vi "子VI-查看某框-不显示界面-只读穿透图模式.vi"(0 "框号":dbl format="%#_13g", 1 "框组":T3(array[cluster]), 2 "临界Z值":i32, 4 "临界面积百分比值":dbl, 5 "预先配置的灰度阈值":dbl, 6 "穿透图原始路径":path, 7 "部位信息":string[](array[string])=["", "34.500000", "32.500000", "1121", "34", "54.955926", "分层类", "不合格", ""], 12 "产品规格":cluster{"产品长度（周长）（mm）":dbl, "产品宽度（母线长）（mm）":dbl}) -> (17 "全部检测结果":string[][](table))   [LabVIEW 2018]
uses:
  <vilib>/vision/NI_Vision_Development_Module.lvlib
panel:
  out "?":string[][](table)
  out "弥散类检测结果":string[][](table)
  in  "格式字符串 4":string="%f"
  in  "分隔符（'\\'代码显示） 3":string="\t"
  in  "Tab Control":T1
  out "?":T2(plugin-control)
  out "Threshold Image":T2(plugin-control)
  out "Threshold Image":T2(plugin-control)
  in  "格式字符串 3":string="%f"
  in  "分隔符（'\\'代码显示） 2":string="\t"
  out "弥散和分层临界灰度值":i64
  out "弥散缺陷个数":i32
  out "分层缺陷个数":i32
  out "合格？ 弥散类":string="fencengThreshold"
  out "合格？分层类":string="fencengThreshold"
  out "弥散测量结果":i16[][](array[numeric])
  out "面积 (pixels)":i32
  in  "格式字符串 2":string="%f"
  in  "分隔符（'\\'代码显示）":string="\t"
  out "分层测量结果":i16[][](array[numeric])
  out "缺陷初步分类的临界值":sgl format="%#.3f"
  # "所选区域信息"
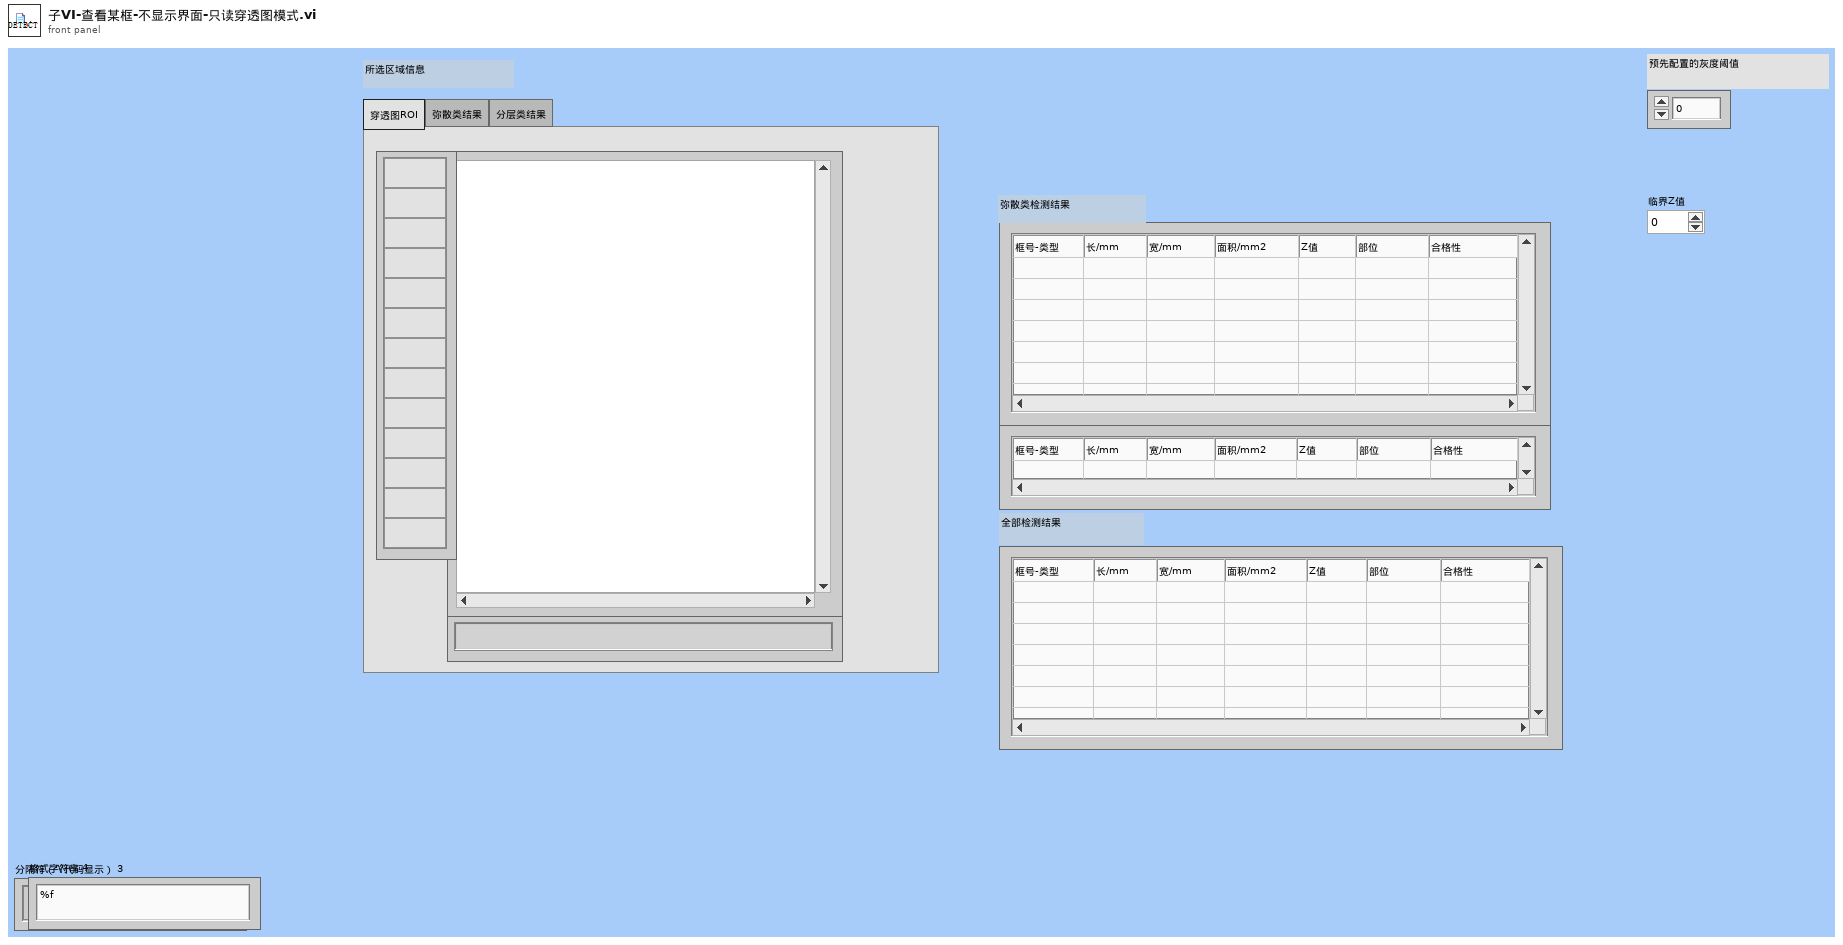
[diagram p1: front panel]
types:
  T1 = typedef "控件2.ctl" = enum32{"穿透图ROI", "弥散类结果", "分层类结果"}
  T2 = typedef "IMAQ Image.ctl" = refnum<image>
  T3 = cluster{"Global Rectangle":i32[], "Contours":cluster{"Contour Type":u32, "ROI Type":u32, "Points":i32[]}[]}[]
  T4 = typedef "Image Type" = u32
  T5 = typedef "Particle Parameters" = i32
  T6 = cluster{"Measurement Parameter":T5, "Range Lower Value":dbl, "Range Upper Value":dbl, "Range":bool, "Measurement Type":bool}[]
  T7 = cluster{"Global Rectangle":i32[], "Contours":cluster{"Contour Type":u32, "ROI Type":u32, "Points":i32[]}[]}
  T8 = cluster{"histogram":u32[], "Minimal Value":sgl, "Maximal Value":sgl, "Starting Value":sgl, "Interval Width":sgl, "Mean Value":sgl, "Standard  Variation":sgl, "Area (pixels)":i32}
  T9 = cluster{"Area":dbl, "Number of Holes":dbl, "Bounding Rect":cluster{"Left":dbl, "Top":dbl, "Right":dbl, "Bottom":dbl}, "Center of Mass":cluster{"X":dbl, "Y":dbl}, "Orientation":dbl, "Dimensions":cluster{"Width":dbl, "Height":dbl}}[]
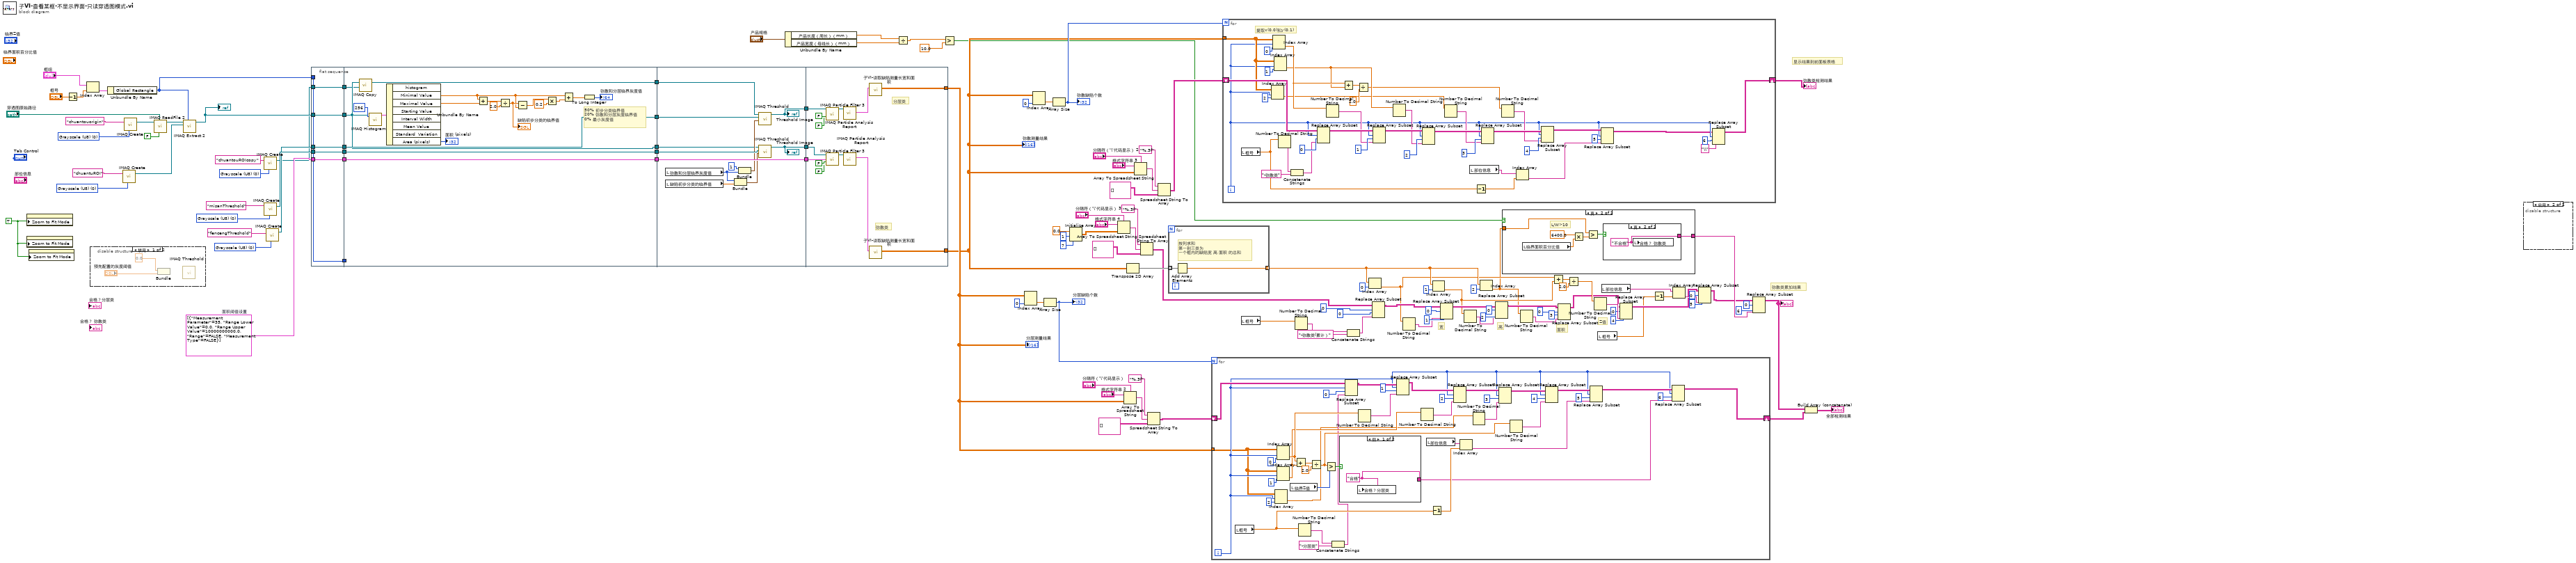
[diagram p0: block diagram]
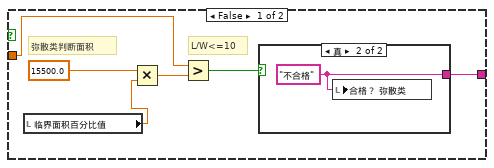
[diagram p2: hidden frame]
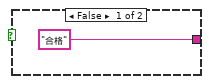
[diagram p3: hidden frame]
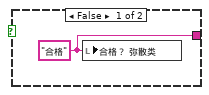
[diagram p4: hidden frame]
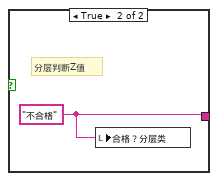
[diagram p6: hidden frame]
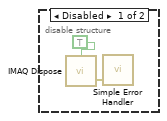
[diagram p7: hidden frame]
diagram:
  w61 = T4 0 items=["Grayscale (U8)", "Grayscale (I16)", "Grayscale (SGL)", "Complex (CSG)", "RGB (U32)", "HSL (U32)", "RGB (U64)", "Grayscale (U16)"] ("Image Type")
  w66 = TRUE ("Zoom to Fit Mode")
  w102 = T4 0 items=["Grayscale (U8)", "Grayscale (I16)", "Grayscale (SGL)", "Complex (CSG)", "RGB (U32)", "HSL (U32)", "RGB (U64)", "Grayscale (U16)"] ("Image Type")
  w103 = T4 0 items=["Grayscale (U8)", "Grayscale (I16)", "Grayscale (SGL)", "Complex (CSG)", "RGB (U32)", "HSL (U32)", "RGB (U64)", "Grayscale (U16)"] ("Image Type")
  w106 = T4 0 items=["Grayscale (U8)", "Grayscale (I16)", "Grayscale (SGL)", "Complex (CSG)", "RGB (U32)", "HSL (U32)", "RGB (U64)", "Grayscale (U16)"] ("Image Type")
  w86 = T6 [{"Measurement Parameter"=35, "Range Lower Value"=0.0, "Range Upper Value"=10000000000.0, "Range"=FALSE, "Measurement Type"=FALSE}]  # 面积阈值设置
  w119 = T4 0 items=["Grayscale (U8)", "Grayscale (I16)", "Grayscale (SGL)", "Complex (CSG)", "RGB (U32)", "HSL (U32)", "RGB (U64)", "Grayscale (U16)"] ("Image Type")
  # "Z值"
  # "面积"
  # "高"
  # "宽"
  # "弥散类累加结果"
  # "显示结果到前面板表格"
  n1 = property class="ImageControl"("Zoom to Fit Mode"=w66) -> ()  [unwired: 2 in, 2 out]
  n2 = property class="ImageControl"("Zoom to Fit Mode"=w66) -> ()  [unwired: 2 in, 2 out]
  n3 = property class="ImageControl"("Zoom to Fit Mode"=w66) -> ()  [unwired: 2 in, 2 out]
  n4 = Decrement(x="框号") -> (x-1=w121:dbl)
  n5 = Index Array(array="框组", index=w121) -> (element=w122:T7)
  n6 = disable-structure shown="禁用" {
    frame Disabled {
      n7 = Bundle(0.0, "预先配置的灰度阈值"="预先配置的灰度阈值") -> ()  [unwired: 1 in, 1 out]
      n8 = call "IMAQ Threshold"() -> ()  [unwired: 6 in, 6 out]
    }
    frame Enabled {
    }
  }
  n9 = Unbundle By Name(w122) -> ("Global Rectangle"=w97:i32[])
  n10 = call "IMAQ Create"("Image Name"="chuantuROI", "Image Type"=w106) -> ("New Image"=w105:T2)  [unwired: 3 in, 1 out]
  n11 = call "IMAQ Create"("Image Name"="chuantouorigin", "Image Type"=w119) -> ("New Image"=w108:T2)  [unwired: 3 in, 1 out]
  n12 = call "IMAQ ReadFile 2"("Use File Path Image Type"=FALSE, "File Path"="穿透图原始路径", "Image"=w108) -> ("Image Out"=w109:T2)  [unwired: 4 in, 4 out]
  n13 = call "IMAQ Extract 2"("Optional Rectangle"=w97, "Image Dst"=w105, "Image Src"=w109) -> ("Image Dst Out"=w69:T2)  [unwired: 7 in, 1 out]
  "?" <- w69
  n14 = call "IMAQ Create"("Image Name"="chuantouROIcopy", "Image Type"=w61) -> ("New Image"=w64:T2)  [unwired: 3 in, 1 out]
  n15 = call "IMAQ Create"("Image Name"="misanThreshold", "Image Type"=w102) -> ("New Image"=w93:T2)  [unwired: 3 in, 1 out]
  n16 = call "IMAQ Create"("Image Name"="fencengThreshold", "Image Type"=w103) -> ("New Image"=w91:T2)  [unwired: 3 in, 1 out]
  n17 = flat-sequence {
    tunnel: w97 -> [w132]
    tunnel: w69 -> [w128]
    tunnel: [w132] -> w96
    tunnel: w93 -> [w131]
    tunnel: [w131] -> w94
    tunnel: [w130] -> w92
    tunnel: w91 -> [w130]
    tunnel: [w129] -> w87
    tunnel: w86 -> [w129]
    tunnel: [w128] -> w67
    tunnel: w64 -> [w127]
    tunnel: [w127] -> w63
    tunnel: [w151] -> w95
    tunnel: [w150] -> w90
    tunnel: [w145] -> w85
    tunnel: w87 -> [w145]
    tunnel: w92 -> [w150]
    tunnel: w94 -> [w151]
    tunnel: w96 -> [_]
    tunnel: [w135] -> w68
    tunnel: w67 -> [w135]
    tunnel: [w134] -> w65
    tunnel: w63 -> [w133]
    tunnel: w95 -> [w163]
    tunnel: w90 -> [w162]
    tunnel: [w153] -> w89
    tunnel: [w154] -> w88
    tunnel: w85 -> [w161]
    tunnel: [w161] -> w84
    tunnel: w68 -> [w155]
    tunnel: w65 -> [w152]
    tunnel: [w166] -> w51
    tunnel: [w167] -> w77
    tunnel: w89 -> [w170]
    tunnel: w88 -> [w171]
    tunnel: w84 -> [w174]
    frame #0 {
    }
    frame #1 {
      # "50% 初步分类临界值\n20% 弥散和分层灰度临界值\n0% 最小灰度值"
      n18 = call "IMAQ Copy"("Image Dst"=w133, "Image Src"=w135) -> ("Image Dst Out"=w134:T2)  [unwired: 4 in, 1 out]
      n19 = call "IMAQ Histogram"("Number of Classes"=256, "Image"=w135) -> ("Histogram Report"=w148:T8)  [unwired: 8 in, 1 out]
      n20 = Unbundle By Name(w148) -> ("Minimal Value"=w137:sgl, "Maximal Value"=w143:sgl, "Area (pixels)"=→"面积 (pixels)":i32)  [unwired: 5 out]
      n21 = Add(x=w137, y=w143) -> (x+y=w142:sgl)
      n22 = Divide(x=w142, y=sgl 2.0) -> (x/y=w141:sgl)
      "缺陷初步分类的临界值" <- w141
      n23 = Subtract(x=w141, y=w137) -> (x-y=w139:sgl)
      n24 = Multiply(x=w139, y=0.2) -> (x*y=w138:dbl)
      n25 = Add(x=w137, y=w138) -> (x+y=w136:dbl)
      n26 = To Long Integer(number=w136) -> (32bit integer=→"弥散和分层临界灰度值":i32)
    }
    frame #2 {
      n27 = local read "弥散和分层临界灰度值"() -> (w157:i64)
      n28 = local read "缺陷初步分类的临界值"() -> (w159:sgl)
      n29 = Bundle("弥散和分层临界灰度值"=w157, "缺陷初步分类的临界值"=w159) -> (w160:cluster{"弥散和分层临界灰度值":i64, "缺陷初步分类的临界值":sgl})  [unwired: 1 in]
      n30 = Bundle(1, "弥散和分层临界灰度值"=w157) -> (w156:cluster{i32, "弥散和分层临界灰度值":i64})  [unwired: 1 in]
      n31 = call "IMAQ Threshold"("Range"=w156, "Image Dst"=w162, "Image Src"=w152) -> ("Image Dst Out"=w153:T2)  [unwired: 3 in, 5 out]
      "Threshold Image" <- w153
      n32 = call "IMAQ Threshold"("Range"=w160, "Image Dst"=w163, "Image Src"=w155) -> ("Image Dst Out"=w154:T2)  [unwired: 3 in, 5 out]
      "Threshold Image" <- w154
    }
    frame #3 {
      # "分层类"
      # "弥散类"
      n33 = call "IMAQ Particle Filter 3"("Image Src"=w170, "Keep/Remove Particles (F)"=FALSE, "Reject Border? (F)"=FALSE) -> ("Image Dst Out"=w169:T2)  [unwired: 10 in, 2 out]
      n34 = call "IMAQ Particle Filter 3"("Image Src"=w171, "Selection Values"=w174, "Keep/Remove Particles (F)"=FALSE, "Reject Border? (F)"=FALSE) -> ("Image Dst Out"=w164:T2)  [unwired: 9 in, 2 out]
      n35 = call "IMAQ Particle Analysis Report"("Image"=w169) -> ("Particle Reports (Pixels)"=w168:T9)  [unwired: 5 in, 5 out]
      n36 = call "IMAQ Particle Analysis Report"("Image"=w164) -> ("Particle Reports (Pixels)"=w165:T9)  [unwired: 5 in, 5 out]
      n37 = call "子VI-读取缺陷测量长宽和面积.vi"("Particle Reports (Pixels)"=w168) -> ("测量结果"=w167:dbl[][])  [unwired: 10 in]
      n38 = call "子VI-读取缺陷测量长宽和面积.vi"("Particle Reports (Pixels)"=w165) -> ("测量结果"=w166:dbl[][])  [unwired: 10 in]
    }
  }
  n39 = Unbundle By Name("产品规格") -> ("产品长度（周长）（mm）"=w113:dbl, "产品宽度（母线长）（mm）"=w112:dbl)
  n40 = Divide(x=w113, y=w112) -> (x/y=w116:dbl)
  n41 = Greater?(x=w116, y=10.0) -> (0:w9:bool)
  n42 = Index Array(array=w77, index (col)=0 ("禁用的索引 (列)")) -> (element=w101:dbl[])  [unwired: 1 in]
  n43 = Index Array(array=w51, index (col)=0 ("禁用的索引 (列)")) -> (element=w99:dbl[])  [unwired: 1 in]
  n44 = Array Size(array=w101) -> (size(s)=w83:i32)
  "分层缺陷个数" <- w83
  n45 = Array Size(array=w99) -> (size(s)=w111:i32)
  "弥散缺陷个数" <- w111
  n46 = Initialize Array(0.0 ("元素"), 1 ("维数大小"), 7 ("维数大小")) -> (w52:dbl[][])
  n47 = Array To Spreadsheet String(delimiter (Tab)="分隔符（'\\'代码显示） 3", array=w52, 3:"格式字符串 4") -> (spreadsheet string=w55:string)
  n48 = Array To Spreadsheet String(delimiter (Tab)="分隔符（'\\'代码显示）", array=w77, 3:"格式字符串 2") -> (spreadsheet string=w80:string)
  n49 = Transpose 2D Array(2D array=w51) -> (transposed array=w50:dbl[][])
  n50 = Array To Spreadsheet String(delimiter (Tab)="分隔符（'\\'代码显示） 2", array=w51, 3:"格式字符串 3") -> (spreadsheet string=w73:string)
  n51 = Spreadsheet String To Array(format string="%.3f", spreadsheet string=w55, array type (2D Dbl)=string[][] [] ("Array")) -> (array=w8:string[][])  [unwired: 1 in]
  n52 = Spreadsheet String To Array(format string="%.3f", spreadsheet string=w80, array type (2D Dbl)=string[][] [] ("Array")) -> (array=w76:string[][])  [unwired: 1 in]
  n53 = Spreadsheet String To Array(format string="%.3f", spreadsheet string=w73, array type (2D Dbl)=string[][] [] ("Array")) -> (array=w70:string[][])  [unwired: 1 in]
  n54 = for {
    tunnel: w50 -> [w178] mode=indexing
    tunnel: [w177] -> w12 mode=indexing
    # "按列求和 \n第一到三类为\n一个框内的缺陷宽 高 面积 的总和"
    n55 = Add Array Elements(numeric array=w178) -> (sum=w177:dbl)
  }
  n56 = for {
    N: w83 -> [_]
    tunnel: w77 -> [w180]
    shift-right: [w193] -> w3
    shift-left: w76 -> [w202]
    i -> [w181]
    n57 = local read "框号"() -> (w209:dbl)
    n58 = Index Array(array=w180, index (row)=w181, index (col)=2 ("索引 (列)")) -> (element=w179:dbl)
    n59 = Index Array(array=w180, index (row)=w181, index (col)=0 ("禁用的索引 (列)")) -> (element=w192:dbl)
    n60 = Index Array(array=w180, index (row)=w181, index (col)=1 ("禁用的索引 (列)")) -> (element=w191:dbl)
    n61 = local read "临界Z值"() -> (w216:i32)
    n62 = Add(x=w192, y=w191) -> (x+y=w217:dbl)
    n63 = Number To Decimal String(number=w209) -> (decimal integer string=w185:string)  [unwired: 1 in]
    n64 = Divide(x=w217, y=2.0) -> (x/y=w189:dbl)
    n65 = Greater?(x=w189, y=w216) -> (0:w218:bool)
    n66 = Concatenate Strings(w185, "-分层类" ("新元素/子数组")) -> (w184:string)
    n67 = case shown="假" w218 {
      tunnel: [w219 w220] -> w187
      frame False {
        w219 = "合格" ("合格？")
        n68 = local write "合格？分层类"(w219) -> ()
      }
      frame True {
        w220 = "不合格" ("合格？")
        # "分层判断Z值"
        n69 = local write "合格？分层类"(w220) -> ()
      }
    }
    n70 = Replace Array Subset(array=w202, new element=w184, index (row)=w181, index (col)=0 ("索引 (列)")) -> (w201:string[][])
    n71 = Number To Decimal String(number=w192) -> (decimal integer string=w200:string)  [unwired: 1 in]
    n72 = Replace Array Subset(array=w201, new element=w200, index (row)=w181, index (col)=1 ("索引 (列)")) -> (w198:string[][])
    n73 = Number To Decimal String(number=w191) -> (decimal integer string=w199:string)  [unwired: 1 in]
    n74 = local read "部位信息"() -> (w212:string[])
    n75 = Decrement(x=w209) -> (x-1=w211:dbl)
    n76 = Replace Array Subset(array=w198, new element=w199, index (row)=w181, index (col)=2 ("索引 (列)")) -> (w197:string[][])
    n77 = Index Array(array=w212, index=w211) -> (element=w188:string)
    n78 = Number To Decimal String(number=w179) -> (decimal integer string=w196:string)  [unwired: 1 in]
    n79 = Replace Array Subset(array=w197, new element=w196, index (row)=w181, index (col)=3 ("索引 (列)")) -> (w195:string[][])
    n80 = Number To Decimal String(number=w189) -> (decimal integer string=w190:string)  [unwired: 1 in]
    n81 = Replace Array Subset(array=w195, new element=w190, index (row)=w181, index (col)=4 ("索引 (列)")) -> (w194:string[][])
    n82 = Replace Array Subset(array=w194, new element=w188, index (row)=w181, index (col)=5 ("索引 (列)")) -> (w183:string[][])
    n83 = Replace Array Subset(array=w183, new element=w187, index (row)=w181, index (col)=6 ("索引 (列)")) -> (w193:string[][])
  }
  n84 = for {
    N: w111 -> [_]
    tunnel: w51 -> [w226]
    shift-right: [w243] -> w5
    shift-left: w70 -> [w249]
    i -> [w224]
    # "提取x(0,0)和y(0,1)"
    n85 = local read "框号"() -> (w231:dbl)
    n86 = Index Array(array=w226, index (row)=w224, index (col)=2 ("禁用的索引 (列)")) -> (element=w223:dbl)
    n87 = Index Array(array=w226, index (row)=w224, index (col)=0 ("禁用的索引 (列)")) -> (element=w237:dbl)
    n88 = Index Array(array=w226, index (row)=w224, index (col)=1 ("禁用的索引 (列)")) -> (element=w236:dbl)
    n89 = Number To Decimal String(number=w231) -> (decimal integer string=w228:string)  [unwired: 1 in]
    n90 = Concatenate Strings(w228, "-弥散类" ("新元素/子数组")) -> (w227:string)
    n91 = Replace Array Subset(array=w249, new element=w227, index (row)=w224, index (col)=0 ("索引 (列)")) -> (w248:string[][])
    n92 = Number To Decimal String(number=w237) -> (decimal integer string=w242:string)  [unwired: 1 in]
    n93 = Add(x=w237, y=w236) -> (x+y=w239:dbl)
    n94 = Divide(x=w239, y=2.0) -> (x/y=w235:dbl)
    n95 = Replace Array Subset(array=w248, new element=w242, index (row)=w224, index (col)=1 ("索引 (列)")) -> (w247:string[][])
    n96 = Number To Decimal String(number=w236) -> (decimal integer string=w241:string)  [unwired: 1 in]
    n97 = Replace Array Subset(array=w247, new element=w241, index (row)=w224, index (col)=2 ("索引 (列)")) -> (w246:string[][])
    n98 = Number To Decimal String(number=w223) -> (decimal integer string=w240:string)  [unwired: 1 in]
    n99 = local read "部位信息"() -> (w233:string[])
    n100 = Decrement(x=w231) -> (x-1=w232:dbl)
    n101 = Replace Array Subset(array=w246, new element=w240, index (row)=w224, index (col)=3 ("索引 (列)")) -> (w245:string[][])
    n102 = Number To Decimal String(number=w235) -> (decimal integer string=w234:string)  [unwired: 1 in]
    n103 = Index Array(array=w233, index=w232) -> (element=w230:string)
    n104 = Replace Array Subset(array=w245, new element=w234, index (row)=w224, index (col)=4 ("索引 (列)")) -> (w244:string[][])
    n105 = Replace Array Subset(array=w244, new element=w230, index (row)=w224, index (col)=5 ("索引 (列)")) -> (w222:string[][])
    n106 = Replace Array Subset(array=w222, new element="\\" ("新元素/子数组"), index (row)=w224, index (col)=6 ("索引 (列)")) -> (w243:string[][])
  }
  "弥散类检测结果" <- w5
  n107 = local read "框号"() -> (w7:dbl)
  n108 = Number To Decimal String(number=w7) -> (decimal integer string=w16:string)  [unwired: 1 in]
  n109 = Concatenate Strings(w16, "-弥散类(累计）" ("新元素/子数组")) -> (w14:string)
  n110 = Index Array(array=w12, index=0 ("索引")) -> (element=w11:dbl)
  n111 = Replace Array Subset(array=w8, new element=w14, index (row)=0 ("禁用的索引 (行)"), index (col)=0 ("索引 (列)")) -> (w44:string[][])
  n112 = Number To Decimal String(number=w11) -> (decimal integer string=w43:string)  [unwired: 1 in]
  n113 = Index Array(array=w12, index=1 ("索引")) -> (element=w10:dbl)
  n114 = Replace Array Subset(array=w44, new element=w43, index (row)=0 ("索引 (行)"), index (col)=1 ("索引 (列)")) -> (w41:string[][])
  n115 = Number To Decimal String(number=w10) -> (decimal integer string=w34:string)  [unwired: 1 in]
  n116 = Index Array(array=w12, index=2 ("索引")) -> (element=w6:dbl)
  n117 = Replace Array Subset(array=w41, new element=w34, index (row)=0 ("索引 (行)"), index (col)=2 ("禁用的索引 (列)")) -> (w36:string[][])
  n118 = case shown="真" w9 {
    tunnel: [w263 w271] -> w17
    tunnel: w6 -> [w259 w267]
    frame False {
      # "弥散类判断面积"
      # "L/W<=10"
      n119 = local read "临界面积百分比值"() -> (w260:dbl)
      n120 = Multiply(x=15500.0, y=w260) -> (x*y=w261:dbl)
      n121 = Greater?(x=w259, y=w261) -> (0:w264:bool)
      n122 = case shown="真" w264 {
        tunnel: ["合格" ("合格？") w266] -> w263
        frame False {
        }
        frame True {
          w266 = "不合格" ("合格？")
          n123 = local write "合格？ 弥散类"(w266) -> ()
        }
      }
    }
    frame True {
      # "L/W>10"
      n124 = local read "临界面积百分比值"() -> (w268:dbl)
      n125 = Multiply(x=6400.0, y=w268) -> (x*y=w270:dbl)
      n126 = Greater?(x=w267, y=w270) -> (0:w272:bool)
      n127 = case shown="真" w272 {
        tunnel: [w273 w274] -> w271
        frame False {
          w273 = "合格" ("合格？")
          n128 = local write "合格？ 弥散类"(w273) -> ()
        }
        frame True {
          w274 = "不合格" ("合格？")
          n129 = local write "合格？ 弥散类"(w274) -> ()
        }
      }
    }
  }
  n130 = Number To Decimal String(number=w6) -> (decimal integer string=w33:string)  [unwired: 1 in]
  n131 = Add(x=w11, y=w10) -> (x+y=w32:dbl)
  n132 = Replace Array Subset(array=w36, new element=w33, index (row)=0 ("索引 (行)"), index (col)=3 ("索引 (列)")) -> (w26:string[][])
  n133 = Divide(x=w32, y=2.0) -> (x/y=w30:dbl)
  n134 = Number To Decimal String(number=w30) -> (decimal integer string=w29:string)  [unwired: 1 in]
  n135 = local read "框号"() -> (w1:dbl)
  n136 = local read "部位信息"() -> (w24:string[])
  n137 = Replace Array Subset(array=w26, new element=w29, index (row)=0 ("索引 (行)"), index (col)=4 ("索引 (列)")) -> (w20:string[][])
  n138 = Decrement(x=w1) -> (x-1=w25:dbl)
  n139 = Index Array(array=w24, index=w25) -> (element=w23:string)
  n140 = Replace Array Subset(array=w20, new element=w23, index (row)=0 ("索引 (行)"), index (col)=5 ("索引 (列)")) -> (w13:string[][])
  n141 = Replace Array Subset(array=w13, new element=w17, index (row)=0 ("索引 (行)"), index (col)=6 ("索引 (列)")) -> (w2:string[][])
  "?" <- w2
  n142 = Build Array (concatenate)(w2, w3) -> (→"全部检测结果":string[][])
  n143 = disable-structure shown="启用" {
    frame Disabled {
      n144 = call "IMAQ Dispose"("All Images? (No)"=TRUE) -> ("error out"=w276:errorcluster)  [unwired: 5 in]
      n145 = call <vilib>:"Simple Error Handler.vi"("error in (no error)"=w276) -> ()  [unwired: 4 in, 5 out]
    }
    frame Enabled {
    }
  }
  "分层测量结果" <- w77
  "弥散测量结果" <- w51
